vi "Modify Run-Time Menu for Spectral Graph.vi"(7 "octave info":T1[](array[typedef]) {"engineering units" items=["custom..."=0, "V"=1, "A"=21, "C"=30, "pC"=31, "s"=32, "-"=29, "Pa"=2, "N"=20, "g"=3, "m/s^2"=4, "m/s"=5, "m"=6, "mm/s"=12, "mm"=13, "micron/s"=14, "micron"=15, "in/s^2"=7, "in/s"=8, "in"=9, "mil/s"=10, "mil"=11, "rad/s^2"=16, "rad/s"=17, "rad"=18, "deg/s^2"=26, "deg/s"=27, "deg"=28, "RPM"=22, "cycle/s^2"=23, "Hz"=24, "cycle"=25, "strain"=19]; "dB reference" format="%.2e"; "weighting filter" items=["Linear", "A-weighting", "B-weighting", "C-weighting", "ITU-R 468-4", "Dolby", "CCITT", "C-message", "Wb", "Wc", "Wd", "We", "Wf", "Wh", "Wj", "Wk", "Wm", "AES17 20 kHz lowpass", "AES17 40 kHz lowpass", "AES17 20 kHz highpass", "AES17 40 kHz highpass"]}, 10 "Menu in":refnum<k9>, 11 "Display State In":T5={"Graph Visible Items"={"Plot Legend"=FALSE, "Scale Legend"=FALSE, "Graph Palette"=FALSE, "Cursor Legend"=FALSE, "X Scrollbar"=FALSE}, "View Table"=FALSE, "Table Visible Items"={"Vertical Scrollbar"=FALSE, "Horizontal Scrollbar"=FALSE, "Row Headers"=FALSE, "Column Headers"=FALSE, "Vertical Lines"=FALSE, "Horizontal Lines"=FALSE}, "Header Font"={"Font Name"="", "Size"=0, "Bold"=FALSE, "Italic"=FALSE, "Underline"=FALSE, "Strikeout"=FALSE, "Color"=0}, "Cell Font"={"Font Name"="", "Size"=0, "Bold"=FALSE, "Italic"=FALSE, "Underline"=FALSE, "Strikeout"=FALSE, "Color"=0}, "Description and Tip..."={"Description"="", "Tip"=""}, "Moveable Splitter Position"=0, "Measurement Cursor Configuration"={"XY"={"enable XY"=FALSE, "Position (X)"=[], "Type"=enum."Absolute", "Y reference"=0.0, "color"=0}, "band"={"enable band"=FALSE, "B1"=0.0, "B2"=0.0, "Fixed bandwidth (B2-B1)"=0.0, "B1 color"=0, "B2 color"=0}, "harmonic"={"enable harmonics"=FALSE, "X reference (1X)"=0.0, "Maximum"=0, "Subset"=enum."All", "1X color"=0, "MX color"=0}, "sideband"={"enable sideband"=FALSE, "X center (C)"=0.0, "Sidebands"=0, "X spacing (s)"=0.0, "Center color"=0, "Sideband color"=0}}, "Cursors"={"List"=[], "Tags"=[]}, "X Increment"=0.0, "X Scale"={"Label Visible"=FALSE, "Label Text"="", "Mapping Mode"=0, "Format String"=""}, "Y Scale"={"Label Visible"=FALSE, "Label Text"="", "Mapping Mode"=0, "Format String"=""}, "Colors"={"background"=16777215, "major grid"=8355711, "minor grid"=12632256, "font"=0}, "desired spectrum view"={"scaling"={"linear/dB"=enum."no change", "dB reference"=0.0, "power/magnitude"=enum."no change", "view"=enum."no change"}, "spectral density"=enum."no change"}, "Plot Color Wheel"=[3381759, 32768, 982784, 4375295, 13827953, 13457919, 16757522, 4343295, 16728758, 12095254], "Plots"=[], "registered user events"=variant, "Lock 1X to Peak"=FALSE} caption="State" {"Y Scale"."Mapping Mode" items=["Linear", "Logarithmic", "dB"]; "X Scale"."Mapping Mode" items=["Linear", "Logarithmic"]}) -> (3 "Display State out":T5={"Graph Visible Items"={"Plot Legend"=FALSE, "Scale Legend"=FALSE, "Graph Palette"=FALSE, "Cursor Legend"=FALSE, "X Scrollbar"=FALSE}, "View Table"=FALSE, "Table Visible Items"={"Vertical Scrollbar"=FALSE, "Horizontal Scrollbar"=FALSE, "Row Headers"=FALSE, "Column Headers"=FALSE, "Vertical Lines"=FALSE, "Horizontal Lines"=FALSE}, "Header Font"={"Font Name"="", "Size"=0, "Bold"=FALSE, "Italic"=FALSE, "Underline"=FALSE, "Strikeout"=FALSE, "Color"=0}, "Cell Font"={"Font Name"="", "Size"=0, "Bold"=FALSE, "Italic"=FALSE, "Underline"=FALSE, "Strikeout"=FALSE, "Color"=0}, "Description and Tip..."={"Description"="", "Tip"=""}, "Moveable Splitter Position"=0, "Measurement Cursor Configuration"={"XY"={"enable XY"=FALSE, "Position (X)"=[], "Type"=enum."Absolute", "Y reference"=0.0, "color"=0}, "band"={"enable band"=FALSE, "B1"=0.0, "B2"=0.0, "Fixed bandwidth (B2-B1)"=0.0, "B1 color"=0, "B2 color"=0}, "harmonic"={"enable harmonics"=FALSE, "X reference (1X)"=0.0, "Maximum"=0, "Subset"=enum."All", "1X color"=0, "MX color"=0}, "sideband"={"enable sideband"=FALSE, "X center (C)"=0.0, "Sidebands"=0, "X spacing (s)"=0.0, "Center color"=0, "Sideband color"=0}}, "Cursors"={"List"=[], "Tags"=[]}, "X Increment"=0.0, "X Scale"={"Label Visible"=FALSE, "Label Text"="", "Mapping Mode"=0, "Format String"=""}, "Y Scale"={"Label Visible"=FALSE, "Label Text"="", "Mapping Mode"=0, "Format String"=""}, "Colors"={"background"=16777215, "major grid"=8355711, "minor grid"=12632256, "font"=0}, "desired spectrum view"={"scaling"={"linear/dB"=enum."no change", "dB reference"=0.0, "power/magnitude"=enum."no change", "view"=enum."no change"}, "spectral density"=enum."no change"}, "Plot Color Wheel"=[3381759, 32768, 982784, 4375295, 13827953, 13457919, 16757522, 4343295, 16728758, 12095254], "Plots"=[], "registered user events"=variant, "Lock 1X to Peak"=FALSE} caption="State" {"Y Scale"."Mapping Mode" items=["Linear", "Logarithmic", "dB"]; "X Scale"."Mapping Mode" items=["Linear", "Logarithmic"]})   [LabVIEW 2017, in "Octave with Cursors.xctl"]
uses:
  <vilib>/addons/_XControls/Octave with Cursors/Octave with Cursors.xctl
  <vilib>/addons/_XControls/Octave with Cursors/Controls/State.ctl
  <vilib>/Utility/miscctls.llb/LVFontTypeDef.ctl
  <vilib>/addons/_XControls/Octave with Cursors/Controls/Measurement Cursor Configuration.ctl
  <vilib>/addons/_NISVFA/_Shared subVIs/Controls/svc_Octave Info.ctl
  <vilib>/addons/_NISVFA/_Shared subVIs/Controls/svc_Octave Standard.ctl
  <vilib>/addons/_NISVFA/_Shared subVIs/Controls/svc_Weighting Filter Text Ring.ctl
  <vilib>/addons/_NISVFA/_Shared subVIs/Controls/svc_Engineering Units Text Ring.ctl
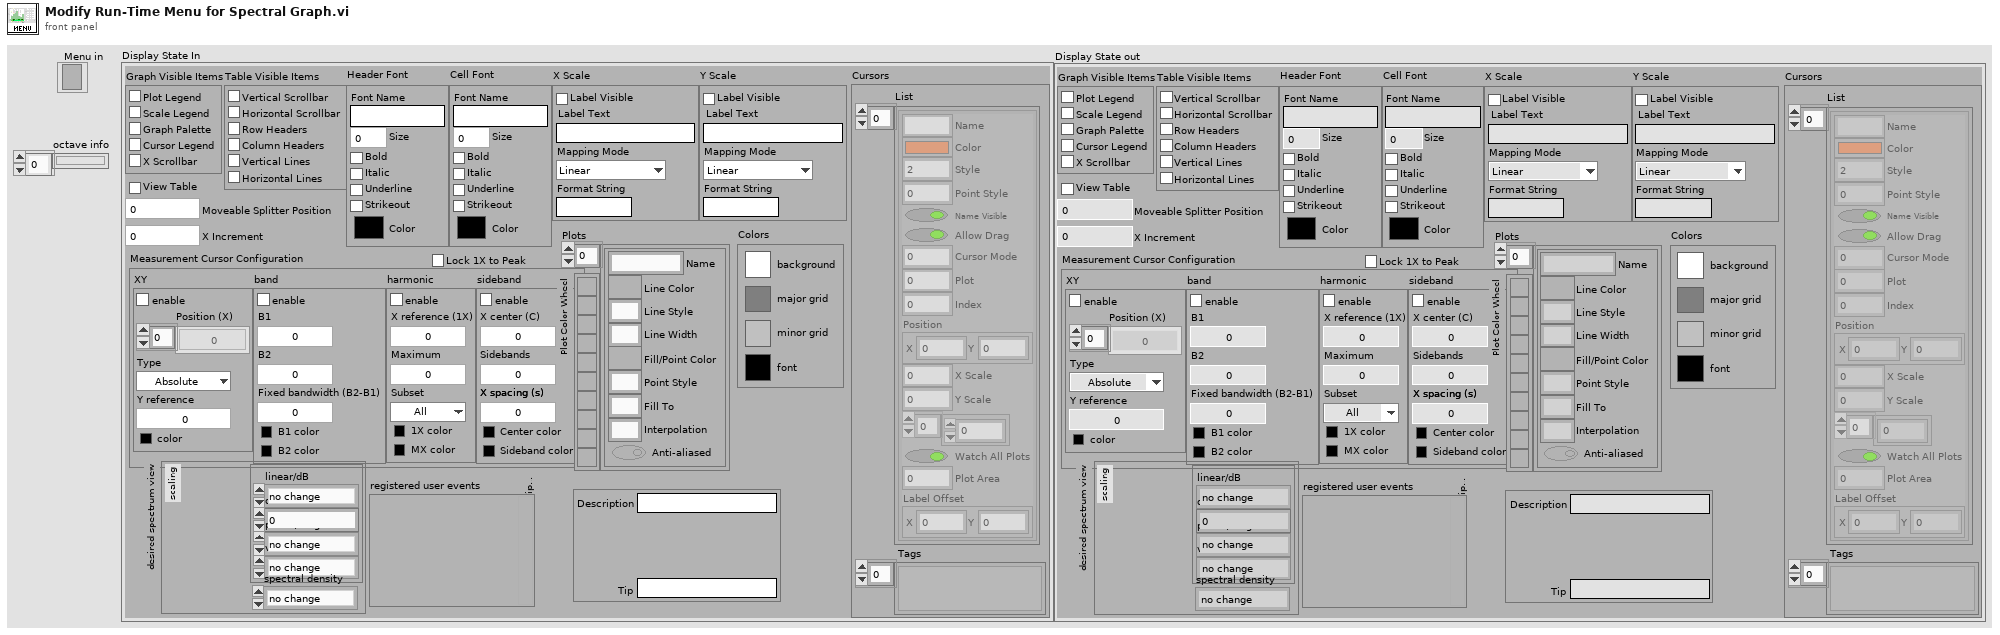
[diagram p1: front panel]
types:
  T1 = typedef "svc_Octave Info.ctl" = cluster{"standard":T2, "bandwidth":enum16{"1 octave", "1/3 octave", "1/6 octave", "1/12 octave", "1/24 octave"}, "low band":i32, "high band":i32, "weighting filter":T3, "dB reference":dbl, "dB On":bool, "unit label":string, "channel name":string, "description":string, "engineering units":T4, "custom label":string, "spectrum type":enum16{"power", "magnitude"}, "spectral density":bool, "filters settled":bool}
  T2 = typedef "svc_Octave Standard.ctl" = enum16{"ANSI S1.11", "IEC 61260"}
  T3 = typedef "svc_Weighting Filter Text Ring.ctl" = u16
  T4 = typedef "svc_Engineering Units Text Ring.ctl" = u16
  T5 = typedef "Octave with Cursors.xctl/State.ctl" = cluster{"Graph Visible Items":cluster{"Plot Legend":bool, "Scale Legend":bool, "Graph Palette":bool, "Cursor Legend":bool, "X Scrollbar":bool}, "View Table":bool, "Table Visible Items":cluster{"Vertical Scrollbar":bool, "Horizontal Scrollbar":bool, "Row Headers":bool, "Column Headers":bool, "Vertical Lines":bool, "Horizontal Lines":bool}, "Header Font":T6, "Cell Font":T6, "Description and Tip...":cluster{"Description":string, "Tip":string}, "Moveable Splitter Position":i32, "Measurement Cursor Configuration":T7, "Cursors":cluster{"List":cluster{"Name":string, "Color":u32, "Style":i32, "Point Style":u8, "Name Visible":bool, "Allow Drag":bool, "Cursor Mode":u32, "Plot":i32, "Index":i32, "Position":cluster{"X":dbl, "Y":dbl}, "X Scale":u32, "Y Scale":u32, "Watch Plots":i32[], "Watch All Plots":bool, "Plot Area":i32, "Label Offset":cluster{"X":dbl, "Y":dbl}}[], "Tags":variant[]}, "X Increment":dbl, "X Scale":cluster{"Label Visible":bool, "Label Text":string, "Mapping Mode":u8, "Format String":string}, "Y Scale":cluster{"Label Visible":bool, "Label Text":string, "Mapping Mode":u8, "Format String":string}, "Colors":cluster{"background":u32, "major grid":u32, "minor grid":u32, "font":u32}, "desired spectrum view":cluster{"scaling":cluster{"linear/dB":enum16{"no change", "linear", "dB"}, "dB reference":dbl, "power/magnitude":enum16{"no change", "power", "magnitude"}, "view":enum16{"no change", "rms", "peak", "peak-peak"}}, "spectral density":enum16{"no change", "spectrum", "spectral density"}}, "Plot Color Wheel":u32[], "Plots":cluster{"Name":string, "Line Color":u32, "Line Style":u8, "Line Width":u8, "Fill/Point Color":u32, "Point Style":u8, "Fill To":i16, "Interpolation":u8, "Anti-aliased":bool}[], "registered user events":variant, "Lock 1X to Peak":bool}
  T6 = typedef "LVFontTypeDef.ctl" = cluster{"Font Name":string, "Size":u16, "Bold":bool, "Italic":bool, "Underline":bool, "Strikeout":bool, "Color":u32}
  T7 = typedef "Octave with Cursors.xctl/Measurement Cursor Configuration.ctl" = cluster{"XY":cluster{"enable XY":bool, "Position (X)":dbl[], "Type":enum16{"Absolute", "Relative"}, "Y reference":dbl, "color":u32}, "band":cluster{"enable band":bool, "B1":dbl, "B2":dbl, "Fixed bandwidth (B2-B1)":dbl, "B1 color":u32, "B2 color":u32}, "harmonic":cluster{"enable harmonics":bool, "X reference (1X)":dbl, "Maximum":i32, "Subset":enum16{"All", "Even", "Odd"}, "1X color":u32, "MX color":u32}, "sideband":cluster{"enable sideband":bool, "X center (C)":dbl, "Sidebands":i32, "X spacing (s)":dbl, "Center color":u32, "Sideband color":u32}}
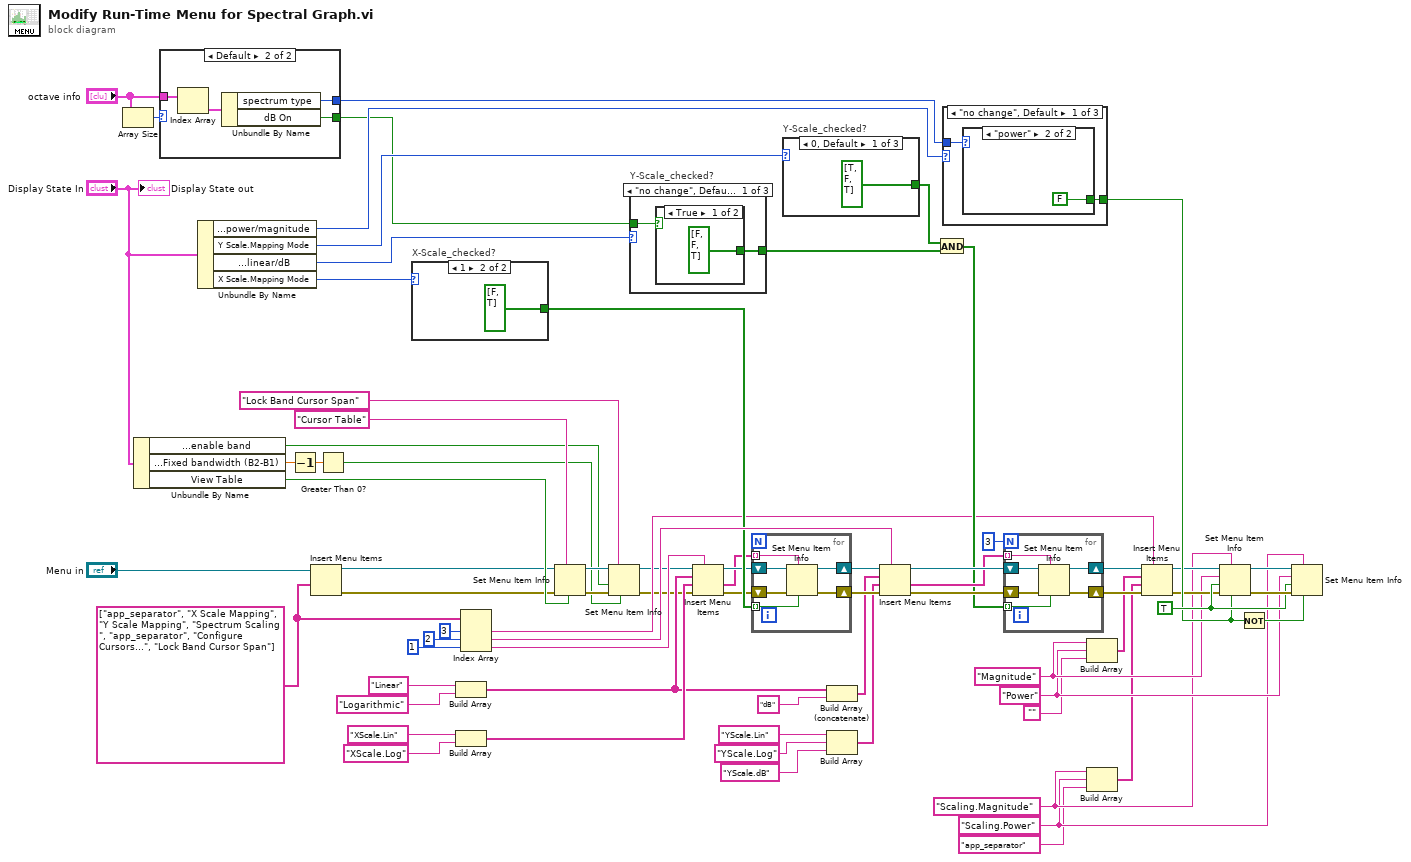
[diagram p0: block diagram]
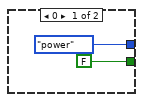
[diagram p2: hidden frame]
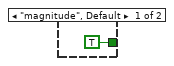
[diagram p3: hidden frame]
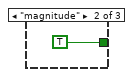
[diagram p4: hidden frame]
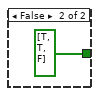
[diagram p6: hidden frame]
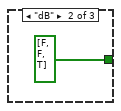
[diagram p7: hidden frame]
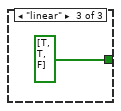
[diagram p8: hidden frame]
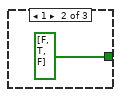
[diagram p9: hidden frame]
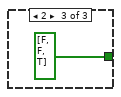
[diagram p10: hidden frame]
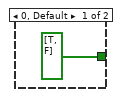
[diagram p11: hidden frame]
diagram:
  w33 = TRUE ("enabled")
  w19 = "Scaling.Power"
  w20 = "Scaling.Magnitude"
  w22 = "Power" ("element")
  w23 = "Magnitude" ("element")
  w67 = string[] ["app_separator", "X Scale Mapping", "Y Scale Mapping", "Spectrum Scaling ", "app_separator", "Configure Cursors...", "Lock Band Cursor Span"]
  n1 = Array Size(array="octave info") -> (size(s)=w15:i32)
  n2 = Unbundle By Name("Display State In") -> ("Measurement Cursor Configuration.band.enable band"=w2:bool, "Measurement Cursor Configuration.band.Fixed bandwidth (B2-B1)"=w6:dbl, "View Table"=w70:bool)
  n3 = case shown="Default" w15 {
    tunnel: "octave info" -> [_ w78]
    tunnel: [enum16{"power", "magnitude"}."power" ("spectrum type") w76] -> w12
    tunnel: [FALSE ("spectral density?") w75] -> w13
    frame 0 {
    }
    frame Default {
      n4 = Index Array(array=w78) -> (element=w77:T1)  [unwired: 1 in]
      n5 = Unbundle By Name(w77) -> ("spectrum type"=w76:enum16{"power", "magnitude"}, "dB On"=w75:bool)
    }
  }
  n6 = Unbundle By Name("Display State In") -> ("desired spectrum view.scaling.power/magnitude"=w32:enum16{"no change", "power", "magnitude"}, "Y Scale.Mapping Mode"=w56:u8, "desired spectrum view.scaling.linear/dB"=w40:enum16{"no change", "linear", "dB"}, "X Scale.Mapping Mode"=w63:u8)
  n7 = Decrement(x=w6) -> (x-1=w1:dbl)
  n8 = Insert Menu Items(7:w67, 9:"Menu in") -> (0:w3:errorcluster, 3:w4:refnum<k9>)  [unwired: 4 in, 1 out]
  n9 = Greater Than 0?(x=w1) -> (x > 0?=w5:bool)
  n10 = case "X-Scale_checked?" shown="1" w63 {
    tunnel: [bool[] [TRUE, FALSE] bool[] [FALSE, TRUE]] -> w55
    frame 0, Default {
    }
    frame 1 {
    }
  }
  n11 = Build Array("Linear", "Logarithmic") -> (w44:string[])
  n12 = Build Array("XScale.Lin", "XScale.Log") -> (w49:string[])
  n13 = Index Array(array=w67, index #1=3 ("index"), index #2=2 ("index"), index #3=1 ("index")) -> (element #1=w24:string, element #2=w64:string, element #3=w52:string)
  n14 = Set Menu Item Info(6:w70, 7:"Cursor Table", 8:w3, 11:w4) -> (0:w11:errorcluster, 3:w10:refnum<k9>)  [unwired: 3 in]
  n15 = Set Menu Item Info(6:w5, 7:"Lock Band Cursor Span", 8:w11, 9:w2, 11:w10) -> (0:w8:errorcluster, 3:w9:refnum<k9>)  [unwired: 2 in]
  n16 = case "Y-Scale_checked?" shown="\"no change\", Default" w40 {
    tunnel: [w82 bool[] [FALSE, FALSE, TRUE] bool[] [TRUE, TRUE, FALSE]] -> w39
    tunnel: w13 -> [w81 _ _]
    frame "no change", Default {
      n17 = case shown="True" w81 {
        tunnel: [bool[] [FALSE, FALSE, TRUE] bool[] [TRUE, TRUE, FALSE]] -> w82
        frame True {
        }
        frame False {
        }
      }
    }
    frame "dB" {
    }
    frame "linear" {
    }
  }
  n18 = Insert Menu Items(5:w52, 6:w8, 7:w49, 8:w44, 9:w9) -> (0:w53:errorcluster, 1:w48:string[], 3:w54:refnum<k9>)  [unwired: 1 in]
  n19 = for {
    shift-right: [w90] -> w61
    shift-left: w54 -> [w92]
    shift-right: [w89] -> w62
    shift-left: w53 -> [w91]
    tunnel: w55 -> [w88] mode=indexing
    tunnel: w48 -> [w87] mode=indexing
    n20 = Set Menu Item Info(6:w88, 7:w87, 8:w91, 11:w92) -> (0:w89:errorcluster, 3:w90:refnum<k9>)  [unwired: 3 in]
  }
  n21 = case "Y-Scale_checked?" shown="0, Default" w56 {
    tunnel: [bool[] [TRUE, FALSE, TRUE] bool[] [FALSE, TRUE, FALSE] bool[] [FALSE, FALSE, TRUE]] -> w37
    frame 0, Default {
    }
    frame 1 {
    }
    frame 2 {
    }
  }
  n22 = Build Array (concatenate)(w44, "dB") -> (w43:string[])
  n23 = Build Array("YScale.Lin", "YScale.Log", "YScale.dB") -> (w45:string[])
  n24 = Insert Menu Items(5:w64, 6:w62, 7:w45, 8:w43, 9:w61) -> (0:w59:errorcluster, 1:w58:string[], 3:w60:refnum<k9>)  [unwired: 1 in]
  n25 = And(x=w37, y=w39) -> (x .and. y?=w38:bool[])
  n26 = case shown="\"no change\", Default" w32 {
    tunnel: [w97 TRUE ("enabled") _] -> w31
    tunnel: w12 -> [w96 _ _]
    frame "no change", Default {
      n27 = case shown="\"power\"" w96 {
        tunnel: [TRUE ("enabled") FALSE ("enabled")] -> w97
        frame "magnitude", Default {
        }
        frame "power" {
        }
      }
    }
    frame "magnitude" {
    }
    frame "power" {
    }
  }
  n28 = for {
    N: 3 -> [_]
    shift-right: [w104] -> w27
    shift-left: w60 -> [w106]
    tunnel: w58 -> [w103] mode=indexing
    shift-right: [w102] -> w28
    shift-left: w59 -> [w105]
    tunnel: w38 -> [w101] mode=indexing
    n29 = Set Menu Item Info(6:w101, 7:w103, 8:w105, 11:w106) -> (0:w102:errorcluster, 3:w104:refnum<k9>)  [unwired: 3 in]
  }
  n30 = Build Array(w23, w22, "" ("element")) -> (w21:string[])
  n31 = Build Array(w20, w19, "app_separator") -> (w18:string[])
  n32 = Insert Menu Items(5:w24, 6:w28, 7:w18, 8:w21, 9:w27) -> (0:w26:errorcluster, 3:w25:refnum<k9>)  [unwired: 1 in, 1 out]
  n33 = Set Menu Item Info(6:w31, 7:w20, 8:w26, 9:w33, 10:w23, 11:w25) -> (0:w34:errorcluster, 3:w35:refnum<k9>)  [unwired: 1 in]
  n34 = Not(x=w31) -> (.not. x?=w30:bool)
  n35 = Set Menu Item Info(6:w30, 7:w19, 8:w34, 9:w33, 10:w22, 11:w35) -> ()  [unwired: 1 in, 2 out]
  "Display State out" <- "Display State In"
